vi "Set Test Settings.vi"(10 "Test Settings":T1, 11 "Start Closed Loop Scan Command in":refnum<class "Start Testing Command.lvclass">) -> (3 "Start Closed Loop Scan Command out":refnum<class "Start Testing Command.lvclass">)   [LabVIEW 2016, in "Start Testing Command.lvclass"]
uses:
  Start Testing Command.lvclass
  Typedefs/TestSettings.ctl
  Start Testing Command.lvclass/Start Testing Command.ctl
  Typedefs/HPMT_Typedefs.lvlib
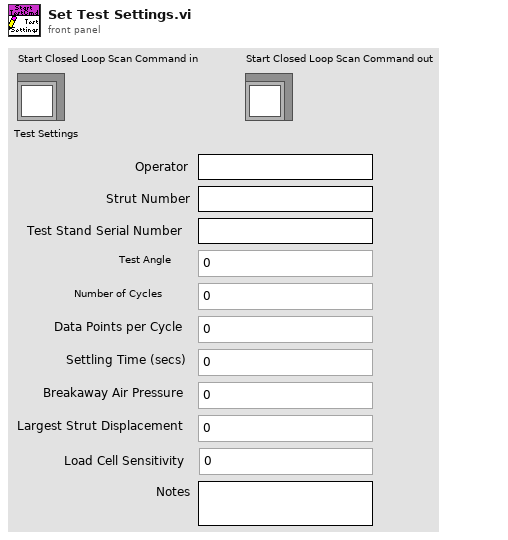
[diagram p1: front panel]
types:
  T1 = typedef "HPMT_Typedefs.lvlib/TestSettings.ctl" = cluster{"Operator":string, "Strut Number":string, "Test Stand Serial Number":string, "Notes":string, "Test Angle":u16, "Number of Cycles":u16, "Data Points per Cycle":u16, "Settling Time (secs)":u16, "Breakaway Air Pressure":u16, "Largest Strut Displacement":dbl, "Load Cell Sensitivity":dbl}
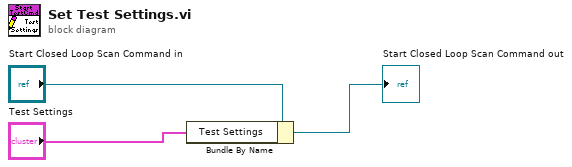
[diagram p0: block diagram]
diagram:
  n1 = Bundle By Name(cluster="Start Closed Loop Scan Command in", "Test Settings"="Test Settings") -> (→"Start Closed Loop Scan Command out":refnum<class "Start Testing Command.lvclass">)
